vi "Broadcast Message.vi"(6 "Timeout ms (1000)":i32=1000, 8 "error in (no error)":errorcluster, 9 "Data":variant, 10 "ID":string, 11 "Basic WebSocket Manager in":refnum<class "Basic WebSocket Manager.lvclass">) -> (0 "error out":errorcluster, 3 "Basic WebSocket Manager out":refnum<class "Basic WebSocket Manager.lvclass">)   [LabVIEW 2020, in "HTTP Server.lvlib" / "Basic WebSocket Manager.lvclass"]
uses:
  Basic WebSocket Manager.lvclass
  ca7e1e62-3144-4158-ac5e-9955634e78aa.vi
  <vilib>/JDP Science/JSONtext/Variant to JSON Text.vi
  <vilib>/JDP Science/JSONtext/LVClass Serializer/JSONtext LVClass Serializer.lvclass
  Basic WebSocket Manager.lvclass/Basic WebSocket Manager.ctl
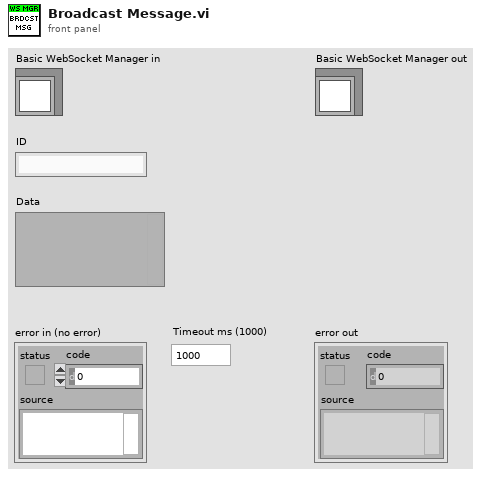
[diagram p1: front panel]
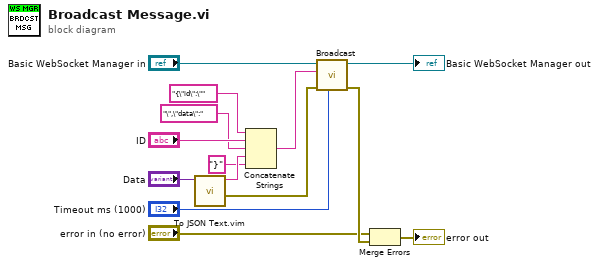
[diagram p0: block diagram]
diagram:
  n1 = call "To JSON Text.vim"("Anything"="Data") -> ("error out"=w3:errorcluster, "<JSON>"=w9:string)  [unwired: 9 in]
  n2 = Concatenate Strings("{\"id\":\"" ("string"), "ID", "\",\"data\":" ("string"), w9, "}" ("string")) -> (w5:string)
  n3 = call "Broadcast.vi"("Timeout ms (1000)"="Timeout ms (1000)", "error in (no error)"=w3, "Payload"=w5, "Basic WebSocket Manager in"="Basic WebSocket Manager in") -> ("error out"=w14:errorcluster, "Basic WebSocket Manager out"=→"Basic WebSocket Manager out":refnum<class "Basic WebSocket Manager.lvclass">)  [unwired: 6 in]
  n4 = Merge Errors("error in (no error)", w14) -> (→"error out":errorcluster)
